vi "Robot Global Data.vi"() -> ()   [LabVIEW 2015]
doc: "This global VI can contain as many global variables as you need. Place a control on the panel, give it a good name. To read or write to it from a VI, drag the icon to the diagram of that VI. You can also drag from the project. Click on the node to change which global you access. You shouldn't have multiple locations writing to a global or it will cause a race-condition."
uses:
  <vilib>/Rock Robotics/WPI/Camera/WPI_CameraImageSize.ctl
  <vilib>/Rock Robotics/WPI/DriverStation/WPI_DriverStationRobotMode2.ctl
  <vilib>/vision/Image Controls.llb/IMAQ Image.ctl
panel:
  out "F Heading":dbl
  out "Heading":dbl
  out "Q W":dbl
  out "Pitch":dbl
  out "Roll":dbl
  out "Yaw":dbl
  out "Q Z":dbl
  out "Q Y":dbl
  out "Q X":dbl
  out "A Z":dbl
  out "A Y":dbl
  out "A X":dbl
  out "D Z":dbl
  out "D Y":dbl
  out "D X":dbl
  out "V Z":dbl
  out "V Y":dbl
  out "V X":dbl
  in  "Masked":T1
  out "Right":dbl
  out "Left":dbl
  in  "E2 Direction":bool
  in  "E1 Direction":bool
  out "E2 Dist":dbl
  out "E1 Dist":dbl
  in  "T3 Visible":bool
  in  "T2 Visible":bool
  in  "T1 Visible":bool
  out "T3 Y":dbl
  out "T3 X":dbl
  out "T3 Dist":dbl
  out "T2 Y":dbl
  out "T2 X":dbl
  out "T2 Dist":dbl
  in  "Robot Mode":T2
  out "T1 Y":dbl
  out "T1 X":dbl
  out "T1 Dist":dbl
  out "KOOl":dbl
  out "ms to process":u32
  out "Detected Totes":T3(array[cluster]) {"Normalized Rect"."Numeric 5" format="%#_2g"; "Normalized Rect"."Numeric 3" format="%#_2g"; "Normalized Rect"."Numeric 2" format="%#_2g"; "Normalized Rect"."Numeric" format="%#_2g"}
  in  "image size":T4=enum."320x240"
  in  "Enable Vision":bool
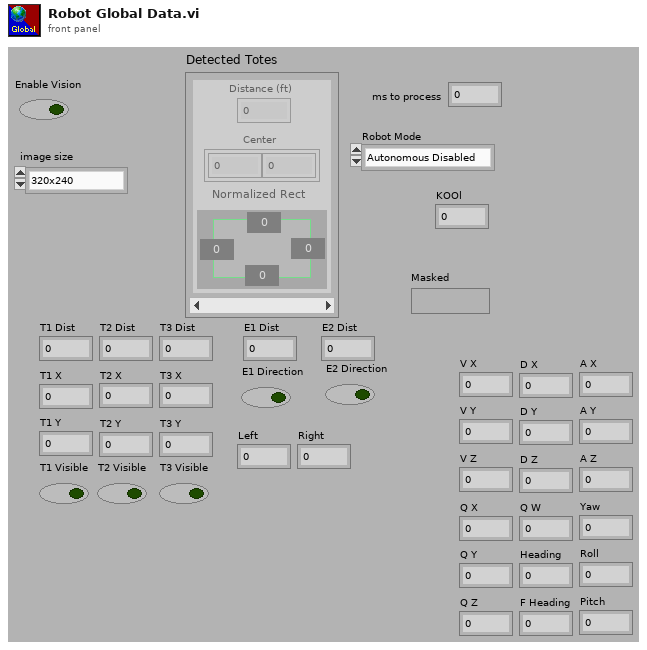
[diagram p1: front panel]
types:
  T1 = typedef "IMAQ Image.ctl" = refnum<image>
  T2 = typedef "WPI_DriverStationRobotMode2.ctl" = enum16{"Autonomous Disabled", "Autonomous Enabled", "Teleop Disabled", "Teleop Enabled", "Disconnected", "Finish", "Test Disabled", "Test Enabled", "Emergency Stopped"}
  T3 = cluster{"Distance (ft)":dbl, "Center":cluster{dbl, dbl}, "Normalized Rect":cluster{"Numeric":dbl, "Numeric 2":dbl, "Numeric 3":dbl, "Numeric 5":dbl}}[]
  T4 = typedef "WPI_CameraImageSize.ctl" = enum16{"640x480", "320x240", "160x120", "Custom"}
diagram:
